vi "Timestamp or now.vi"(1 "timestamp (now)":timestamp) -> (0 "timestamp":timestamp)   [LabVIEW 2019]
doc: "<b>Description</b> Returns the input timestamp or \"now\".\n\n<b>Inputs</b>\n<b>timestamp</b>: An input timestamp or invalid timestamp.\n\n<b>Outputs</b>\n<b>timestamp</b>: Returns the input timestamp it is is valid, or 'now'.\n\nBSD 3-Clause License\n\nCopyright (c) 2021, TauTerra, LLC\nAll rights reserved.\n\nRedistribution and use in source and binary forms, with or without\nmodification, are permitted provided that the following conditions are met:\n\n1. Redistributions of source code must retain the above copyright notice, this\n list of conditions and the following disclaimer.\n\n2. Redistributions in binary form must reproduce the above copyright notice,\n this list of conditions and the following disclaimer in the documentation\n and/or other materials provided with the distribution.\n\n3. Neither the name of the copyright holder nor the names of its\n contributors may be used to endorse or promote products derived from\n this software without specific prior written permission.\n\nTHIS SOFTWARE IS PROVIDED BY THE COPYRIGHT HOLDERS AND CONTRIBUTORS \"AS IS\"\nAND ANY EXPRESS OR IMPLIED WARRANTIES, INCLUDING, BUT NOT LIMITED TO, THE\nIMPLIED WARRANTIES OF MERCHANTABILITY AND FITNESS FOR A PARTICULAR PURPOSE ARE\nDISCLAIMED. IN NO EVENT SHALL THE COPYRIGHT HOLDER OR CONTRIBUTORS BE LIABLE\nFOR ANY DIRECT, INDIRECT, INCIDENTAL, SPECIAL, EXEMPLARY, OR CONSEQUENTIAL\nDAMAGES (INCLUDING, BUT NOT LIMITED TO, PROCUREMENT OF SUBSTITUTE GOODS OR\nSERVICES; LOSS OF USE, DATA, OR PROFITS; OR BUSINESS INTERRUPTION) HOWEVER\nCAUSED AND ON ANY THEORY OF LIABILITY, WHETHER IN CONTRACT, STRICT LIABILITY,\nOR TORT (INCLUDING NEGLIGENCE OR OTHERWISE) ARISING IN ANY WAY OUT OF THE USE\nOF THIS SOFTWARE, EVEN IF ADVISED OF THE POSSIBILITY OF SUCH DAMAGE."
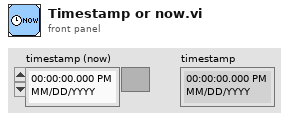
[diagram p1: front panel]
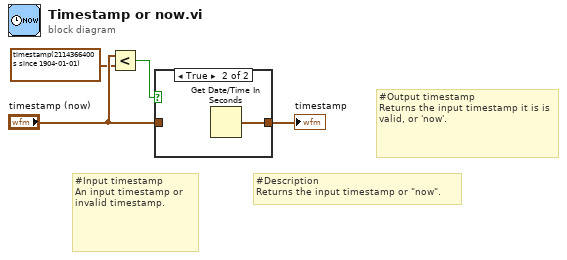
[diagram p0: block diagram]
diagram:
  # "#Output timestamp\nReturns the input timestamp it is is valid, or 'now'."
  # "#Input timestamp\nAn input timestamp or invalid timestamp."
  # "#Description\nReturns the input timestamp or \"now\"."
  n1 = Less?(x="timestamp (now)", y=timestamp(2114366400 s since 1904-01-01) ("timestamp (now)")) -> (x < y?=w2:bool)
  n2 = case shown="True" w2 {
    tunnel: [w5 w6] -> w3
    tunnel: "timestamp (now)" -> [w5 _]
    frame False {
    }
    frame True {
      n3 = Get Date/Time In Seconds() -> (seconds since 1Jan1904=w6:timestamp)
    }
  }
  "timestamp" <- w3
